vi "Example_solar_home_monitoring.vi"() -> ()   [LabVIEW 2023]
uses:
  usbtmc_scpi_labtool.lvlib
panel:
  out "IV Curve of Load":cluster{dbl, dbl}(graph)
  out "IV Curve of PV":cluster{dbl, dbl}(graph)
  in  "stop":bool
  out "Boolean":bool
  in  "VISA resource name in":refnum<visa-resource-name>="USB0::0xCAFE::0x4000::123456::INSTR"
  in  "Load ON/OFF":bool
  out "Load":dbl(slide) scale=0.0..100.0
  out "Charging":u8(slide) scale=0.0..100.0
  out "Load Current":dbl(knob) scale=0.0..30.0
  out "Battery Voltage":dbl(slide) scale=0.0..12.0
  out "Carging Current":dbl
  out "Panel  Voltage":dbl
  out "Charging Current (%)":dbl(knob) scale=0.0..100.0
  out "Panel Voltage (%)":dbl(knob) scale=0.0..100.0
  # "Data from Solar Panel"
  # "Data from Load Side"
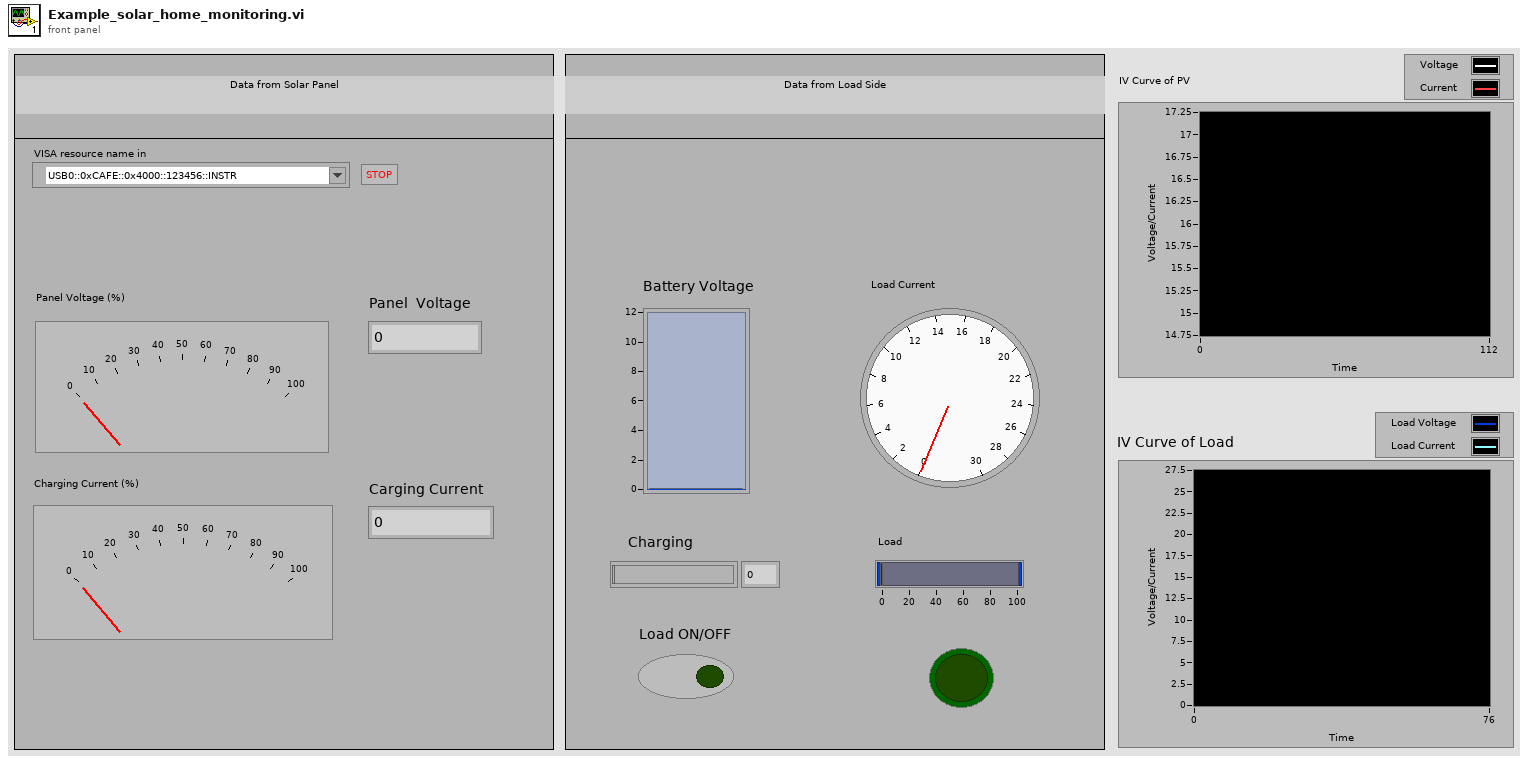
[diagram p1: front panel]
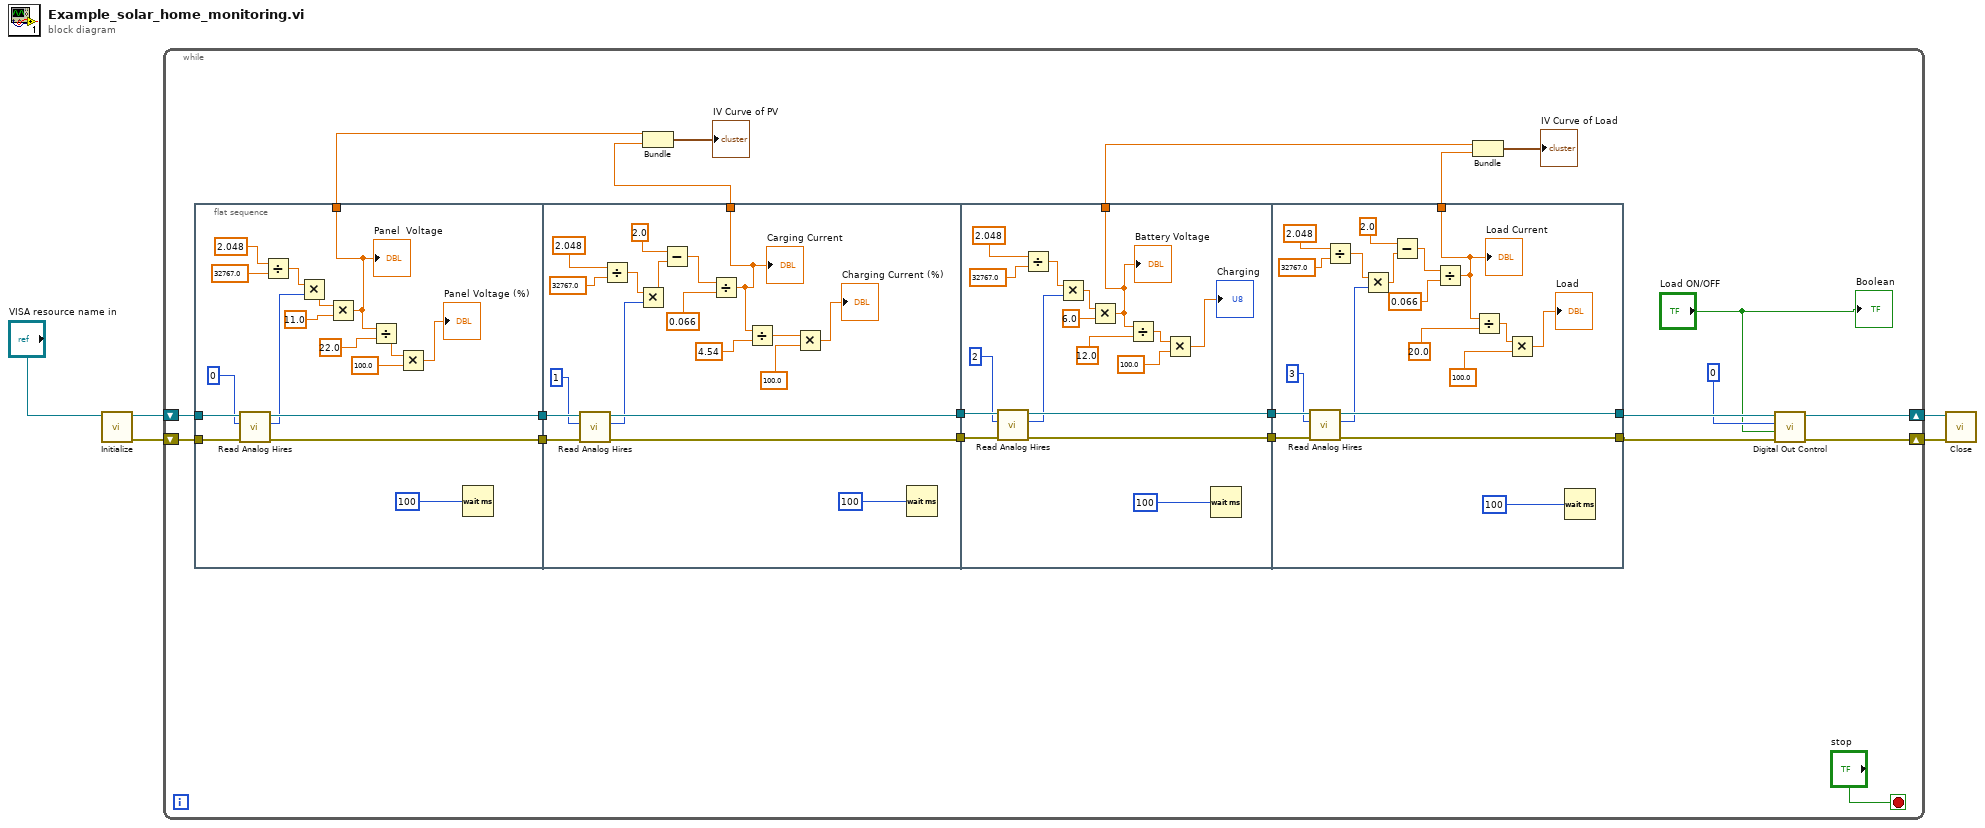
[diagram p0: block diagram]
diagram:
  n1 = call "Initialize.vi"("VISA resource name in"="VISA resource name in") -> ("error out"=w4:errorcluster, "VISA resource name out"=w5:refnum<visa-resource-name>)  [unwired: 9 in]
  n2 = while {
    shift-right: [w11] -> w2
    shift-left: w5 -> [w20]
    shift-right: [w10] -> w3
    shift-left: w4 -> [w19]
    stop <- "stop" stop-if-true
    n3 = flat-sequence {
      tunnel: w20 -> [w43]
      tunnel: w19 -> [w41]
      tunnel: [w42] -> w26
      tunnel: [w40] -> w25
      tunnel: [w27] -> w15
      tunnel: w26 -> [w61]
      tunnel: w25 -> [w62]
      tunnel: [w60] -> w24
      tunnel: [w59] -> w23
      tunnel: [w44] -> w17
      tunnel: w24 -> [w79]
      tunnel: w23 -> [w78]
      tunnel: [w77] -> w22
      tunnel: [w76] -> w21
      tunnel: [w63] -> w14
      tunnel: w22 -> [w98]
      tunnel: w21 -> [w97]
      tunnel: [w96] -> w8
      tunnel: [w95] -> w9
      tunnel: [w80] -> w13
      frame #0 {
        n4 = call "Read Analog Hires.vi"("error in (no error)"=w41, "Pin"=u8 0, "VISA resource name"=w43) -> ("error out"=w40:errorcluster, "analog out"=w35:i32, "VISA resource name out"=w42:refnum<visa-resource-name>)  [unwired: 6 in]
        n5 = Divide(x=2.048, y=32767.0) -> (x/y=w36:dbl)
        n6 = Multiply(x=w36, y=w35) -> (x*y=w34:dbl)
        n7 = Multiply(x=w34, y=11.0) -> (x*y=w27:dbl)
        "Panel  Voltage" <- w27
        n8 = Divide(x=w27, y=22.0) -> (x/y=w31:dbl)
        n9 = Multiply(x=w31, y=100.0) -> (x*y=→"Panel Voltage (%)":dbl)
        n10 = Wait (ms)(milliseconds to wait=u32 100) -> ()  [unwired: 1 out]
      }
      frame #1 {
        n11 = call "Read Analog Hires.vi"("error in (no error)"=w62, "Pin"=u8 1, "VISA resource name"=w61) -> ("error out"=w60:errorcluster, "analog out"=w54:i32, "VISA resource name out"=w59:refnum<visa-resource-name>)  [unwired: 6 in]
        n12 = Divide(x=2.048, y=32767.0) -> (x/y=w55:dbl)
        n13 = Multiply(x=w55, y=w54) -> (x*y=w53:dbl)
        n14 = Subtract(x=2.0, y=w53) -> (x-y=w51:dbl)
        n15 = Divide(x=w51, y=0.066) -> (x/y=w44:dbl)
        "Carging Current" <- w44
        n16 = Divide(x=w44, y=4.54) -> (x/y=w48:dbl)
        n17 = Multiply(x=w48, y=100.0) -> (x*y=→"Charging Current (%)":dbl)
        n18 = Wait (ms)(milliseconds to wait=u32 100) -> ()  [unwired: 1 out]
      }
      frame #2 {
        n19 = call "Read Analog Hires.vi"("error in (no error)"=w79, "Pin"=u8 2, "VISA resource name"=w78) -> ("error out"=w77:errorcluster, "analog out"=w71:i32, "VISA resource name out"=w76:refnum<visa-resource-name>)  [unwired: 6 in]
        n20 = Divide(x=2.048, y=32767.0) -> (x/y=w72:dbl)
        n21 = Multiply(x=w72, y=w71) -> (x*y=w70:dbl)
        n22 = Multiply(x=w70, y=6.0) -> (x*y=w63:dbl)
        "Battery Voltage" <- w63
        n23 = Divide(x=w63, y=12.0) -> (x/y=w67:dbl)
        n24 = Multiply(x=w67, y=100.0) -> (x*y=→"Charging":dbl)
        n25 = Wait (ms)(milliseconds to wait=u32 100) -> ()  [unwired: 1 out]
      }
      frame #3 {
        n26 = call "Read Analog Hires.vi"("error in (no error)"=w98, "Pin"=u8 3, "VISA resource name"=w97) -> ("error out"=w96:errorcluster, "analog out"=w90:i32, "VISA resource name out"=w95:refnum<visa-resource-name>)  [unwired: 6 in]
        n27 = Divide(x=2.048, y=32767.0) -> (x/y=w91:dbl)
        n28 = Multiply(x=w91, y=w90) -> (x*y=w89:dbl)
        n29 = Subtract(x=2.0, y=w89) -> (x-y=w87:dbl)
        n30 = Divide(x=w87, y=0.066) -> (x/y=w80:dbl)
        "Load Current" <- w80
        n31 = Divide(x=w80, y=20.0) -> (x/y=w84:dbl)
        n32 = Multiply(x=w84, y=100.0) -> (x*y=→"Load":dbl)
        n33 = Wait (ms)(milliseconds to wait=u32 100) -> ()  [unwired: 1 out]
      }
    }
    n34 = Bundle(w15, w17) -> (→"IV Curve of PV":cluster{dbl, dbl})  [unwired: 1 in]
    n35 = Bundle(w14, w13) -> (→"IV Curve of Load":cluster{dbl, dbl})  [unwired: 1 in]
    n36 = call "Digital Out Control.vi"("VISA resource name"=w9, "Pin"=u8 0, "Enable Pin (F: Off)"="Load ON/OFF", "error in (no error)"=w8) -> ("VISA resource name out"=w11:refnum<visa-resource-name>, "error out"=w10:errorcluster)  [unwired: 5 in]
    "Boolean" <- "Load ON/OFF"
  }
  n37 = call "Close.vi"("error in (no error)"=w3, "VISA resource name"=w2) -> ()  [unwired: 10 in]
